vi "Async Message.vi"() -> ()   [LabVIEW 2021, in "Async Methods Actor.lvlib"]
uses:
  Async Methods Actor.lvlib
  Async Methods Actor Messages/Async Message/Async Message.lvclass
panel:
  in  "Async Message":refnum<class "Async Message.lvclass">
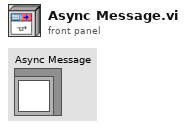
[diagram p1: front panel]
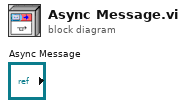
[diagram p0: block diagram]
diagram:
